vi "get_min_and_max.vi"(8 "error in (no error)":errorcluster, 11 "ImageCollection in":refnum<class "ImageCollection.lvclass">) -> (0 "error out":errorcluster, 1 "minimum":dbl, 2 "maximum":dbl, 3 "ImageCollection out":refnum<class "ImageCollection.lvclass">, 4 "range":dbl)   [LabVIEW 2010, in "ImageCollection.lvclass"]
uses:
  ImageCollection.lvclass
  Image/Image/Image.lvclass
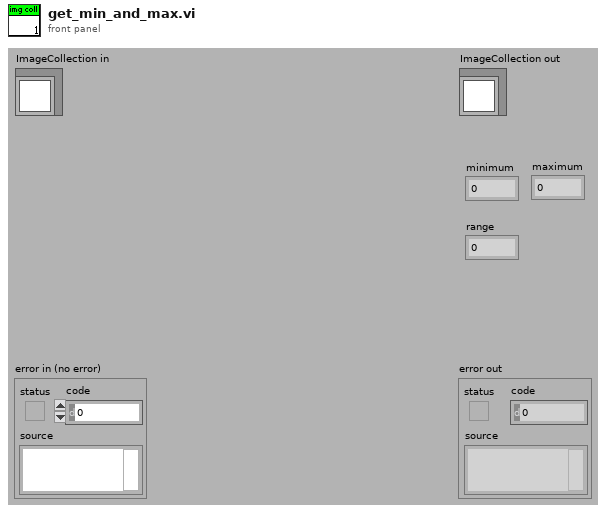
[diagram p1: front panel]
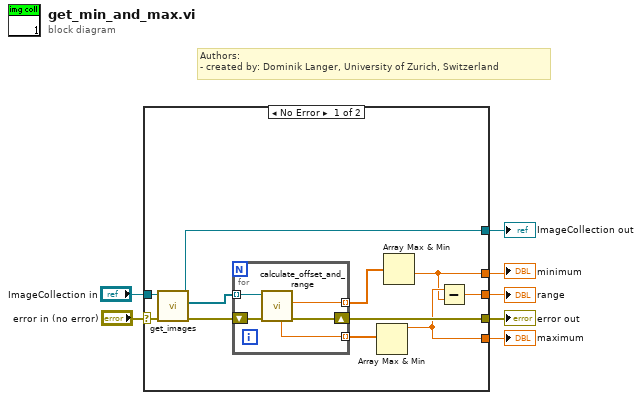
[diagram p0: block diagram]
diagram:
  # "Authors: \n- created by: Dominik Langer, University of Zurich, Switzerland"
  n1 = case shown="No Error" "error in (no error)" {
    selector: "error in (no error)" -> [w17 w25]
    tunnel: [w18 w25] -> w6
    tunnel: [w12 w24] -> w4
    tunnel: "ImageCollection in" -> [w13 w24]
    tunnel: [w9 _] -> w3
    tunnel: [w8 _] -> w2
    tunnel: [w14 _] -> w1
    frame No Error {
      n2 = call-dynamic "get_images.vi"("error in (no error)"=w17, "ImageCollection.lvclass in"=w13) -> ("error out"=w16:errorcluster, "images"=w15:refnum<class "Image.lvclass">[], "ImageCollection.lvclass out"=w12:refnum<class "ImageCollection.lvclass">)  [unwired: 7 in]
      n3 = for {
        shift-right: [w21] -> w18
        shift-left: w16 -> [w23]
        tunnel: w15 -> [w22] mode=indexing
        tunnel: [w20] -> w11 mode=indexing
        tunnel: [w19] -> w10 mode=indexing
        n4 = call-dynamic "calculate_offset_and_range.vi"("error in (no error)"=w23, "Image in"=w22) -> ("error out"=w21:errorcluster, "offset / minimum"=w20:dbl, "maximum"=w19:dbl)  [unwired: 5 in, 2 out]
      }
      n5 = Array Max & Min(array=w10) -> (max value=w9:dbl)  [unwired: 3 out]
      n6 = Array Max & Min(array=w11) -> (min value=w8:dbl)  [unwired: 3 out]
      n7 = Subtract(x=w9, y=w8) -> (x-y=w14:dbl)
    }
    frame Error {
    }
  }
  "error out" <- w6
  "ImageCollection out" <- w4
  "range" <- w1
  "maximum" <- w3
  "minimum" <- w2
